vi "User Console Interface.vi"(7 "Command":T2, 8 "error in (no error)":errorcluster, 10 "Parameter":variant) -> (0 "error out":errorcluster, 1 "timed out?":bool, 2 "Parameter Out":variant caption="Parameter", 3 "User Input":T1 caption="Command")   [LabVIEW 2011]
uses:
  TypeDefs/User Console Commands.ctl
  TypeDefs/UI to CTRL Command.ctl
  TypeDefs/CTRL to UI Message.ctl
  TypeDefs/CTRL to UI Command.ctl
  TypeDefs/UI to CTRL Message.ctl
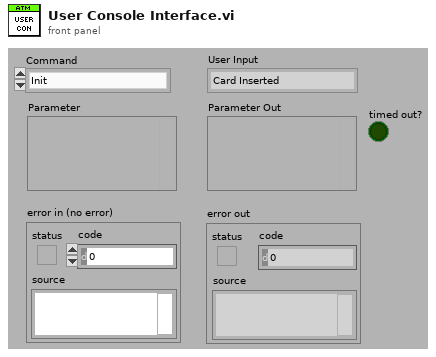
[diagram p1: front panel]
types:
  T1 = typedef "UI to CTRL Command.ctl" = enum16{"Card Inserted", "Keypad Entry", "Button Pressed"}
  T2 = typedef "User Console Commands.ctl" = enum16{"Init", "Set ATM Message", "Set ATM Menus", "Disable Controls", "Wait for Input", "Clear Keypad", "Return Card", "Close"}
  T3 = typedef "UI to CTRL Message.ctl" = cluster{"Command":T1, "Data":variant}
  T4 = typedef "CTRL to UI Message.ctl" = cluster{"Command":T5, "Data":variant}
  T5 = typedef "CTRL to UI Command.ctl" = enum16{"Display Message", "Return Card", "Stop", "Set Menu", "Clear Keypad", "Disable UI Elements"}
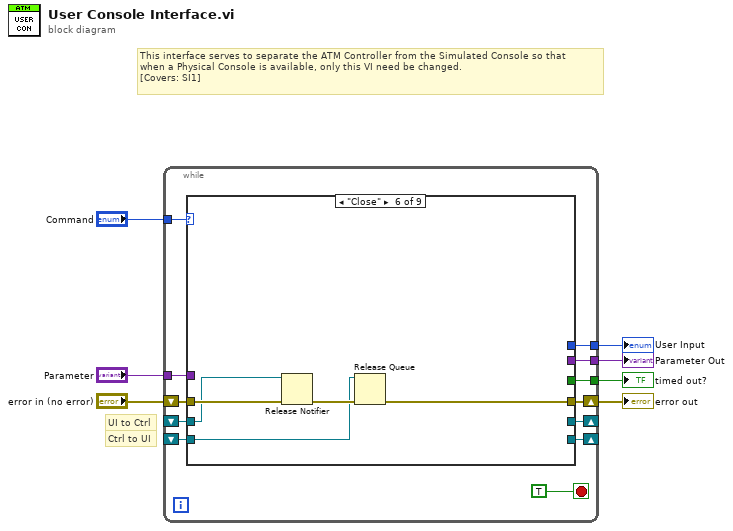
[diagram p0: block diagram]
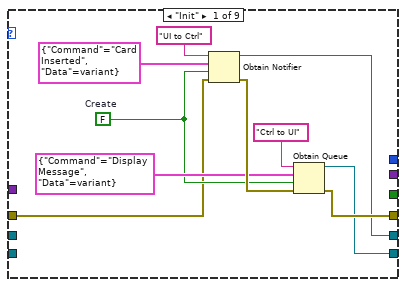
[diagram p2: hidden frame]
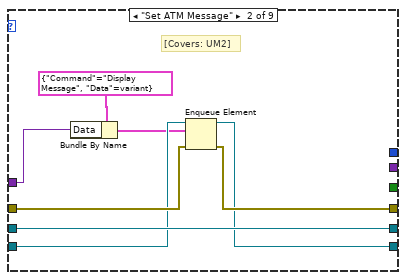
[diagram p3: hidden frame]
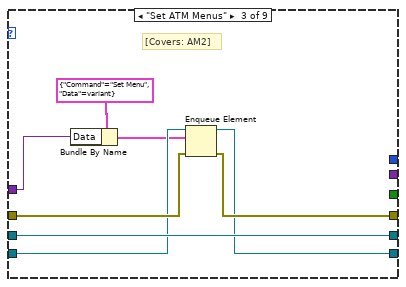
[diagram p4: hidden frame]
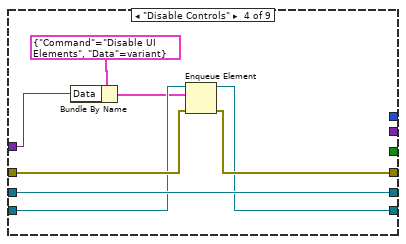
[diagram p5: hidden frame]
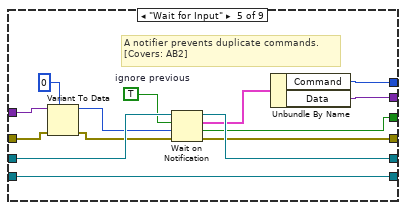
[diagram p6: hidden frame]
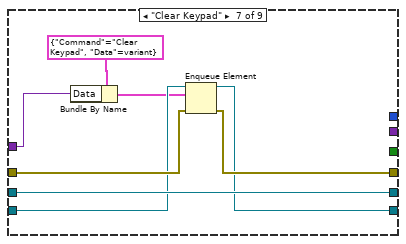
[diagram p7: hidden frame]
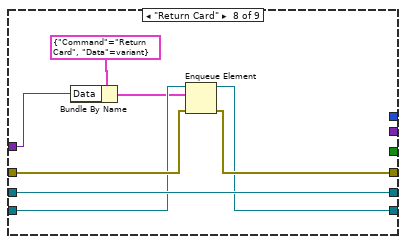
[diagram p8: hidden frame]
diagram:
  # "Ctrl to UI"
  # "UI to Ctrl"
  # "This interface serves to separate the ATM Controller from the Simulated Console so that\nwhen a Physical Console is available, only this VI need be changed.\n[Covers: SI1]"
  n1 = while {
    tunnel: "Command" -> [w18]
    shift-right: [w16] -> w5
    shift-left: "error in (no error)" -> [w17]
    shift-right: [w15] -> _
    shift-left: _ -> [w13]
    shift-right: [w14] -> _
    shift-left: _ -> [w12]
    tunnel: "Parameter" -> [w11]
    tunnel: [w10] -> w3
    tunnel: [w9] -> w2
    tunnel: [w8] -> w1
    stop <- TRUE stop-if-true
    n2 = case shown="\"Close\"" w18 {
      tunnel: w17 -> [w23 w36 w44 w52 w58 w72 w79 w87 w90]
      tunnel: [w22 w35 w43 w51 w64 w68 w78 w86 w90] -> w16
      tunnel: [w21 w37 w45 w53 w65 _ w80 w88 w92] -> w15
      tunnel: [w20 w33 w41 w49 w67 _ w76 w84 w91] -> w14
      tunnel: w13 -> [_ w37 w45 w53 w66 w71 w80 w88 w92]
      tunnel: w12 -> [_ w34 w42 w50 w67 w69 w77 w85 w91]
      tunnel: w11 -> [_ w31 w39 w47 w59 _ w74 w82 w89]
      tunnel: [_ _ _ _ w62 _ _ _ w89] -> w10
      tunnel: [_ _ _ _ w61 _ _ _ _] -> w9
      tunnel: [_ _ _ _ w54 _ _ _ _] -> w8
      frame "Init" {
        w24 = FALSE  # Create
        n3 = Obtain Notifier(name (unnamed)="UI to Ctrl", notification data type=T3 {"Command"=enum."Card Inserted", "Data"=variant} ("Cluster"), create if not found? (T)=w24, error in (no error)=w23) -> (notifier out=w21:refnum<notifier>, error out=w29:errorcluster)  [unwired: 1 out]
        n4 = Obtain Queue(name (unnamed)="Ctrl to UI", element data type=T4 {"Command"=enum."Display Message", "Data"=variant} ("Cluster"), create if not found? (T)=w24, error in (no error)=w29) -> (queue out=w20:refnum<queue>, error out=w22:errorcluster)  [unwired: 1 in, 1 out]
      }
      frame "Set ATM Message" {
        # "[Covers: UM2]"
        n5 = Bundle By Name(cluster=T4 {"Command"=enum."Display Message", "Data"=variant} ("element"), "Data"=w31) -> (w30:T4)
        n6 = Enqueue Element(queue=w34, element=w30, error in (no error)=w36) -> (queue out=w33:refnum<queue>, error out=w35:errorcluster)  [unwired: 1 in, 1 out]
      }
      frame "Set ATM Menus" {
        # "[Covers: AM2]"
        n7 = Bundle By Name(cluster=T4 {"Command"=enum."Set Menu", "Data"=variant} ("element"), "Data"=w39) -> (w38:T4)
        n8 = Enqueue Element(queue=w42, element=w38, error in (no error)=w44) -> (queue out=w41:refnum<queue>, error out=w43:errorcluster)  [unwired: 1 in, 1 out]
      }
      frame "Disable Controls" {
        n9 = Bundle By Name(cluster=T4 {"Command"=enum."Disable UI Elements", "Data"=variant} ("element"), "Data"=w47) -> (w46:T4)
        n10 = Enqueue Element(queue=w50, element=w46, error in (no error)=w52) -> (queue out=w49:refnum<queue>, error out=w51:errorcluster)  [unwired: 1 in, 1 out]
      }
      frame "Wait for Input" {
        w60 = TRUE  # ignore previous
        # "A notifier prevents duplicate commands.\n[Covers: AB2]"
        n11 = Variant To Data(error in=w58, type=0, Variant=w59) -> (data=w55:i32, error out=w57:errorcluster)
        n12 = Wait on Notification(notifier=w66, ignore previous (F)=w60, timeout in ms (-1)=w55, error in (no error)=w57) -> (notifier out=w65:refnum<notifier>, notification=w63:T3, timed out?=w54:bool, error out=w64:errorcluster)
        n13 = Unbundle By Name(w63) -> ("Command"=w61:T1, "Data"=w62:variant)
      }
      frame "Close" {
        n14 = Release Notifier(notifier=w71, error in (no error)=w72) -> (error out=w70:errorcluster)  [unwired: 1 in, 2 out]
        n15 = Release Queue(queue=w69, error in (no error)=w70) -> (error out=w68:errorcluster)  [unwired: 1 in, 2 out]
      }
      frame "Clear Keypad" {
        n16 = Bundle By Name(cluster=T4 {"Command"=enum."Clear Keypad", "Data"=variant} ("element"), "Data"=w74) -> (w73:T4)
        n17 = Enqueue Element(queue=w77, element=w73, error in (no error)=w79) -> (queue out=w76:refnum<queue>, error out=w78:errorcluster)  [unwired: 1 in, 1 out]
      }
      frame "Return Card" {
        n18 = Bundle By Name(cluster=T4 {"Command"=enum."Return Card", "Data"=variant} ("element"), "Data"=w82) -> (w81:T4)
        n19 = Enqueue Element(queue=w85, element=w81, error in (no error)=w87) -> (queue out=w84:refnum<queue>, error out=w86:errorcluster)  [unwired: 1 in, 1 out]
      }
      frame Default {
        # "Throw a system error indicating enum mistmatch."
      }
    }
  }
  "error out" <- w5
  "User Input" <- w2
  "Parameter Out" <- w3
  "timed out?" <- w1
